vi "Test PQ Multiuser.vi"() -> ()   [LabVIEW 2019, in "LV-Data.PGSQL.lvclass"]
uses:
  LV-Data.PGSQL.lvclass
  API/Read Variable (double).vi
panel:
  out "Value 2":dbl
  out "error out":errorcluster
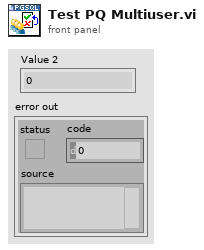
[diagram p1: front panel]
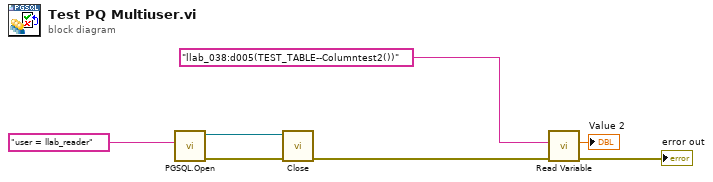
[diagram p0: block diagram]
diagram:
  n1 = call "PGSQL.Open.vi"("Connection String"="user = llab_reader") -> ("error out"=w4:errorcluster, "Data.PG out"=w3:refnum<class "LV-Data.PGSQL.lvclass">)  [unwired: 9 in]
  n2 = call-dynamic "Close.vi"("error in (no error)"=w4, "Data.PG in"=w3) -> ("error out"=w2:errorcluster)  [unwired: 8 in, 1 out]
  n3 = call-poly "Read Variable.vi"("error in (no error)"=w2, "PG path"="llab_038:d005(TEST_TABLE--Columntest2())" ("variable")) -> ("error out"=→"error out":errorcluster, "Value"=→"Value 2":dbl)  [unwired: 4 in, 4 out]
